vi "FromRepo.vi"(8 "error in":errorcluster, 9 "from repo cluster":T2, 10 "repository in":refnum<class "CEF_Repository.lvclass">, 11 "CEF_Node in":refnum<class "CEF_Node.lvclass">) -> (0 "error out":errorcluster, 2 "repository out":refnum<class "CEF_Repository.lvclass">, 3 "node":T1)   [LabVIEW 2025, in "CEF.lvlib" / "CEF_Node.lvclass"]
doc: "Grabs information from the Repo and stores it in the nodes.Copyright 2017 National Instruments Corporation\n\nLicensed under the Apache License, Version 2.0 (the \"License\"); you may not use this file except in compliance with the License. You may obtain a copy of the License at http://www.apache.org/licenses/LICENSE-2.0\nUnless required by applicable law or agreed to in writing, software distributed under the License is distributed on an \"AS IS\" BASIS, WITHOUT WARRANTIES OR CONDITIONS OF ANY KIND, either express or implied. See the License for the specific language governing permissions and limitations under the License."
uses:
  CEF_Node.lvclass
  Repository/CEF_Repository.lvclass
  FromRepoCluster.ctl
  NodeRef.ctl
  CEF_Node.lvclass/CEF_Node.ctl
  WriteParent.vi
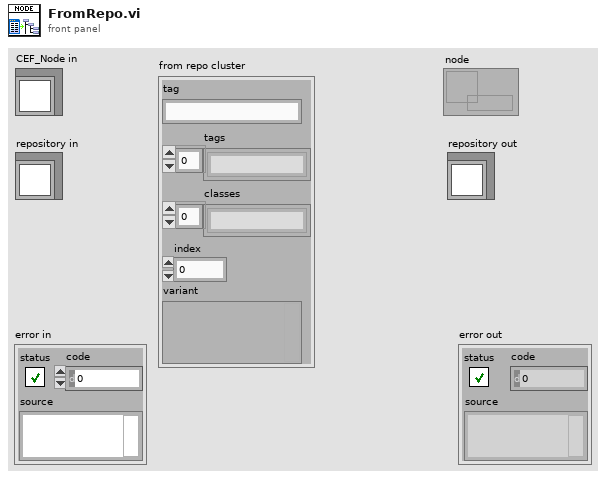
[diagram p1: front panel]
types:
  T1 = typedef "CEF.lvlib/CEF_Node.lvclass/NodeRef.ctl" = refnum<data-value>
  T2 = typedef "CEF.lvlib/CEF_Node.lvclass/FromRepoCluster.ctl" = cluster{"tag":string, "tags":string[], "classes":string[], "index":i32, "variant":variant}
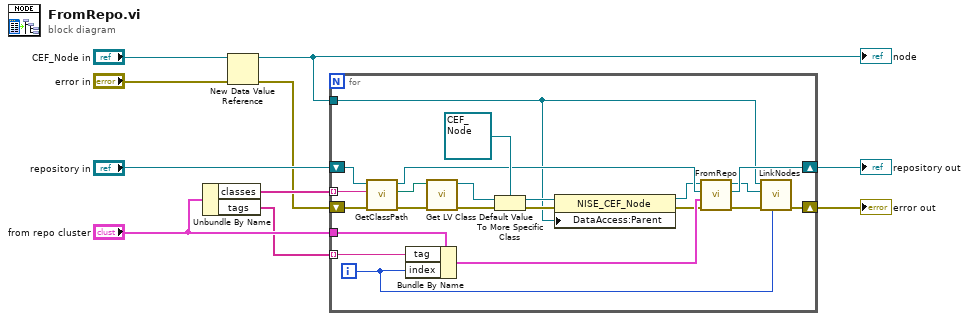
[diagram p0: block diagram]
diagram:
  n1 = Unbundle By Name("from repo cluster") -> ("classes"=w3:string[], "tags"=w2:string[])
  n2 = New Data Value Reference(data value="CEF_Node in", error in="error in") -> (data value reference=w4:refnum<data-value>, error out=w1:errorcluster)
  "node" <- w4
  n3 = for {
    tunnel: w3 -> [w15] mode=indexing
    shift-right: [w28] -> w6
    shift-left: "repository in" -> [w20]
    shift-right: [w25] -> w9
    shift-left: w1 -> [w19]
    tunnel: w4 -> [w11]
    tunnel: w2 -> [w23] mode=indexing
    tunnel: "from repo cluster" -> [w22]
    i -> [w21]
    n4 = call-dynamic "GetClassPath.vi"("error in"=w19, "class name"=w15, "CEF_Repository in"=w20) -> ("error out"=w18:errorcluster, "class path"=w17:path, "CEF_Repository out"=w16:refnum<class "CEF_Repository.lvclass">)  [unwired: 6 in]
    n5 = Bundle By Name(cluster=w22, "tag"=w23, "index"=w21) -> (w24:T2)
    n6 = call <vilib>:"Get LV Class Default Value.vi"("error in (no error)"=w18, "class path"=w17) -> ("error out"=w30:errorcluster, "object"=w31:refnum<class>)  [unwired: 8 in]
    n7 = To More Specific Class(target class=refnum<class "CEF_Node.lvclass"> refnum ("node.lvclass"), reference=w31, error in=w30) -> (specific class reference=w13:refnum<class "CEF_Node.lvclass">, error out=w29:errorcluster)
    n8 = property class="NISE_CEF_Node"(reference=w13, error in=w29, "DataAccess:Parent"=w11) -> (reference out=w12:refnum<class "CEF_Node.lvclass">, error out=w14:errorcluster)
    n9 = call-dynamic "FromRepo.vi"("error in"=w14, "from repo cluster"=w24, "repository in"=w16, "CEF_Node in"=w12) -> ("error out"=w26:errorcluster, "repository out"=w28:refnum<class "CEF_Repository.lvclass">, "node"=w27:T1)  [unwired: 5 in]
    n10 = call "LinkNodes.vi"("index"=w21, "error in"=w26, "child in"=w27, "parent in"=w11) -> ("error out"=w25:errorcluster)  [unwired: 5 in, 2 out]
  }
  "error out" <- w9
  "repository out" <- w6
